vi "Write Message Stream.vi"(10 "Message Stream":refnum<class "Message Stream.lvclass">, 11 "Test in":refnum<class "Test.lvclass">) -> (3 "Test out":refnum<class "Test.lvclass">)   [LabVIEW 2019, in "Test.lvlib" / "Test.lvclass"]
uses:
  Test.lvclass
  <vilib>/ni/Actors/Network Endpoint Actors/Abstract Classes/Message Stream/Message Stream.lvclass
  Test.lvclass/Test.ctl
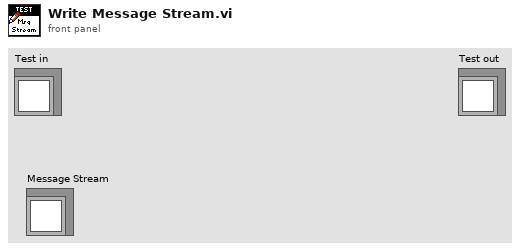
[diagram p1: front panel]
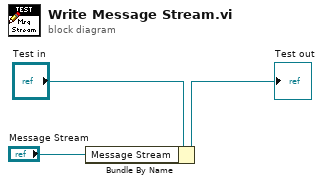
[diagram p0: block diagram]
diagram:
  n1 = Bundle By Name(cluster="Test in", "Message Stream"="Message Stream") -> (→"Test out":refnum<class "Test.lvclass">)
